vi "StepProfileCalc2.vi"(3 "Max speed":dbl, 4 "Move amount":dbl, 5 "Acceleration":dbl, 6 "Step size":dbl) -> (1 "StepTimes":cluster{dbl, "y":dbl}[](array[cluster]), 2 "ActualMovement":dbl)   [LabVIEW 2013]
panel:
  out "Pulse Low Time":dbl format="%#_13g"
  out "Steps needed":dbl
  out "x-y 2":dbl
  out "Numeric":dbl
  out "x-y":dbl
  out "Number of steps":i32
  out "Steps acc":dbl
  out "Dist acc":dbl
  out "Steps needed":dbl
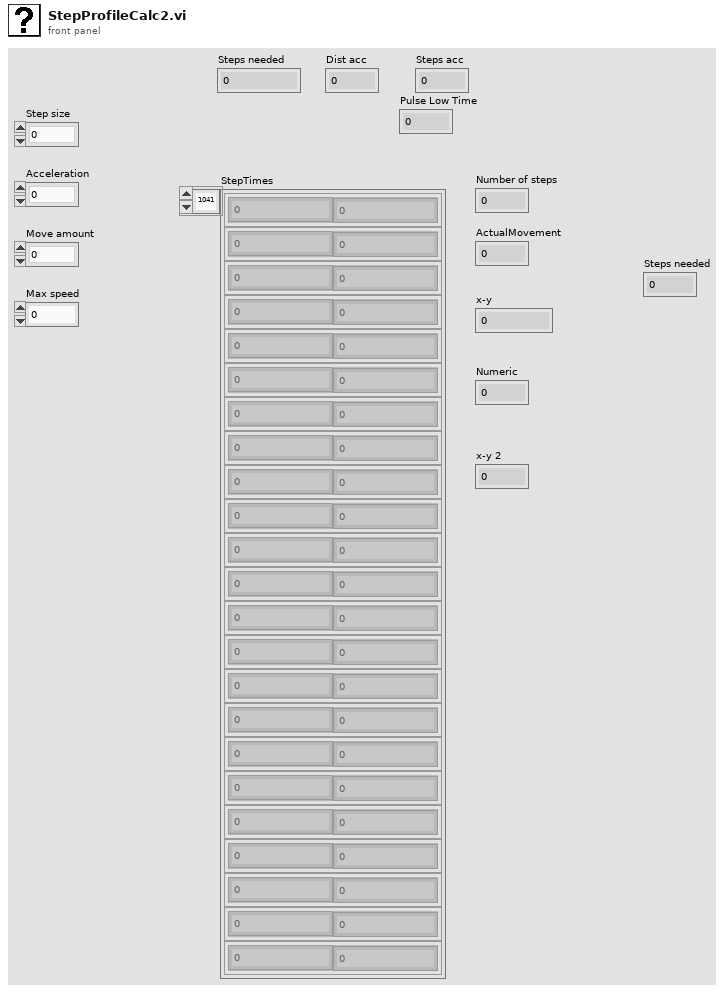
[diagram p1: front panel]
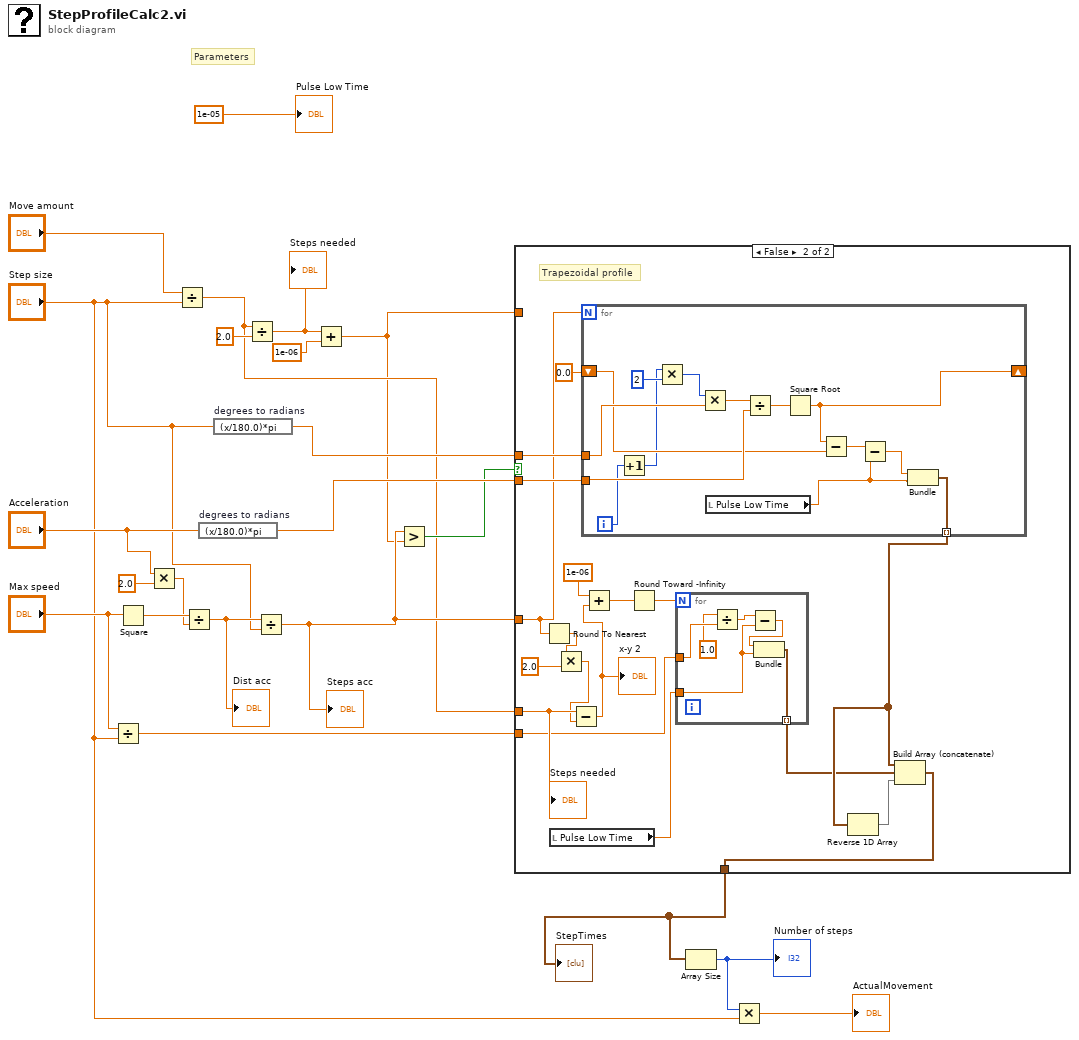
[diagram p0: block diagram]
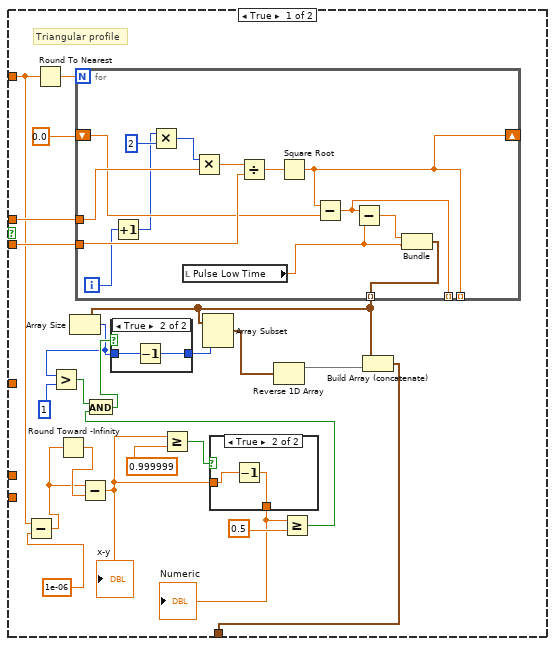
[diagram p2: hidden frame]
diagram:
  # "Parameters"
  n1 = Divide(x="Max speed", y="Step size") -> (x/y=w9:dbl)
  n2 = Square(x="Max speed") -> (x^2=w18:dbl)
  n3 = Multiply(x="Acceleration", y=2.0) -> (x*y=w15:dbl)
  n4 = Divide(x="Move amount", y="Step size") -> (x/y=w11:dbl)
  n5 = Divide(x=w18, y=w15) -> (x/y=w14:dbl)
  "Dist acc" <- w14
  n6 = expression code="(x/180.0)*pi" "degrees to radians"("Acceleration") -> (w20:dbl)
  n7 = expression code="(x/180.0)*pi" "degrees to radians"("Step size") -> (w21:dbl)
  n8 = Divide(x=w11, y=2.0) -> (x/y=w4:dbl)
  "Steps needed" <- w4
  n9 = Divide(x=w14, y="Step size") -> (x/y=w12:dbl)
  "Steps acc" <- w12
  n10 = Add(x=w4, y=1e-06) -> (x+y=w3:dbl)
  n11 = Greater?(x=w12, y=w3) -> (0:w13:bool)
  n12 = case shown="False" w13 {
    tunnel: w3 -> [w30 _]
    tunnel: w21 -> [w45 w83]
    tunnel: w20 -> [w44 w82]
    tunnel: [w28 w77] -> w8
    tunnel: w12 -> [_ w67]
    tunnel: w11 -> [_ w79]
    tunnel: w9 -> [_ w73]
    frame True {
      # "Triangular profile"
      n13 = Subtract(x=w30, y=1e-06) -> (x-y=w31:dbl)
      n14 = Round To Nearest(number=w30) -> (nearest integer value=w40:dbl)
      n15 = Round Toward -Infinity(1:w31) -> (0:w41:dbl)
      n16 = for {
        N: w40 -> [_]
        tunnel: w45 -> [w62]
        tunnel: w44 -> [w61]
        shift-right: [w54] -> _
        shift-left: 0.0 -> [w59]
        tunnel: [w55] -> w37 mode=indexing
        tunnel: [w54] -> _ mode=indexing
        tunnel: [w53] -> _ mode=indexing
        i -> [w58]
        n17 = Increment(x=w58) -> (x+1=w57:i32)
        n18 = Multiply(x=w57, y=2) -> (x*y=w64:i32)
        n19 = local read "Pulse Low Time"() -> (w52:dbl)
        n20 = Multiply(x=w64, y=w62) -> (x*y=w63:dbl)
        n21 = Divide(x=w63, y=w61) -> (x/y=w60:dbl)
        n22 = Square Root(x=w60) -> (sqrt(x)=w54:dbl)
        n23 = Subtract(x=w54, y=w59) -> (x-y=w53:dbl)
        n24 = Subtract(x=w53, y=w52) -> (x-y=w56:dbl)
        n25 = Bundle(w56, "Pulse Low Time"=w52) -> (w55:cluster{dbl, "Pulse Low Time":dbl})  [unwired: 1 in]
      }
      n26 = Array Size(array=w37) -> (size(s)=w33:i32)
      n27 = Greater?(x=w33, y=1) -> (0:w34:bool)
      n28 = Subtract(x=w31, y=w41) -> (x-y=w25:dbl)
      "x-y" <- w25
      n29 = Greater Or Equal?(x=w25, y=0.999999) -> (x >= y?=w23:bool)
      n30 = case shown="True" w23 {
        tunnel: w25 -> [w46 w48]
        tunnel: [w46 w47] -> w26
        frame False {
        }
        frame True {
          n31 = Decrement(x=w48) -> (x-1=w47:dbl)
        }
      }
      "Numeric" <- w26
      n32 = Greater Or Equal?(x=w26, y=0.5) -> (x >= y?=w36:bool)
      n33 = And(x=w34, y=w36) -> (x .and. y?=w35:bool)
      n34 = case shown="True" w35 {
        tunnel: [w49 w51] -> w38
        tunnel: w33 -> [w49 w50]
        frame False {
        }
        frame True {
          n35 = Decrement(x=w50) -> (x-1=w51:i32)
        }
      }
      n36 = Array Subset(array=w37, length=w38) -> (w39:cluster{dbl, "Pulse Low Time":dbl}[])  [unwired: 1 in]
      n37 = Reverse 1D Array(array=w39) -> (reversed array=w42:cluster{dbl, "Pulse Low Time":dbl}[])
      n38 = Build Array (concatenate)(w37, w42) -> (w28:cluster{dbl, "Pulse Low Time":dbl}[])
    }
    frame False {
      # "Trapezoidal profile"
      n39 = Round To Nearest(number=w67) -> (nearest integer value=w68:dbl)
      n40 = local read "Pulse Low Time"() -> (w66:dbl)
      n41 = Multiply(x=w68, y=2.0) -> (x*y=w78:dbl)
      n42 = Subtract(x=w79, y=w78) -> (x-y=w69:dbl)
      "x-y 2" <- w69
      n43 = for {
        N: w67 -> [_]
        tunnel: w83 -> [w100]
        tunnel: w82 -> [w99]
        shift-right: [w96] -> _
        shift-left: 0.0 -> [w97]
        tunnel: [w91] -> w75 mode=indexing
        i -> [w95]
        n44 = Increment(x=w95) -> (x+1=w94:i32)
        n45 = Multiply(x=w94, y=2) -> (x*y=w102:i32)
        n46 = Multiply(x=w102, y=w100) -> (x*y=w101:dbl)
        n47 = local read "Pulse Low Time"() -> (w90:dbl)
        n48 = Divide(x=w101, y=w99) -> (x/y=w98:dbl)
        n49 = Square Root(x=w98) -> (sqrt(x)=w96:dbl)
        n50 = Subtract(x=w96, y=w97) -> (x-y=w93:dbl)
        n51 = Subtract(x=w93, y=w90) -> (x-y=w92:dbl)
        n52 = Bundle(w92, "Pulse Low Time"=w90) -> (w91:cluster{dbl, "Pulse Low Time":dbl})  [unwired: 1 in]
      }
      n53 = Add(x=1e-06, y=w69) -> (x+y=w70:dbl)
      n54 = Round Toward -Infinity(1:w70) -> (0:w72:dbl)
      n55 = for {
        N: w72 -> [_]
        tunnel: [w89] -> w74 mode=indexing
        tunnel: w73 -> [w88]
        tunnel: w66 -> [w84]
        n56 = Divide(x=1.0, y=w88) -> (x/y=w86:dbl)
        n57 = Subtract(x=w86, y=w84) -> (x-y=w85:dbl)
        n58 = Bundle(w85, "Pulse Low Time"=w84) -> (w89:cluster{dbl, "Pulse Low Time":dbl})  [unwired: 1 in]
      }
      n59 = Reverse 1D Array(array=w75) -> (reversed array=w76:cluster{dbl, "Pulse Low Time":dbl}[])
      n60 = Build Array (concatenate)(w75, w74, w76) -> (w77:cluster{dbl, "Pulse Low Time":dbl}[])
      "Steps needed" <- w79
    }
  }
  "StepTimes" <- w8
  n61 = Array Size(array=w8) -> (size(s)=w7:i32)
  "Number of steps" <- w7
  n62 = Multiply(x=w7, y="Step size") -> (x*y=→"ActualMovement":dbl)
  "Pulse Low Time" <- 1e-05 ("y")
